vi "LCD Test.vi"() -> ()   [LabVIEW 2017]
panel:
  in  "stop":bool
  in  "String":string
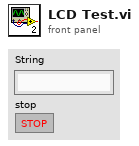
[diagram p1: front panel]
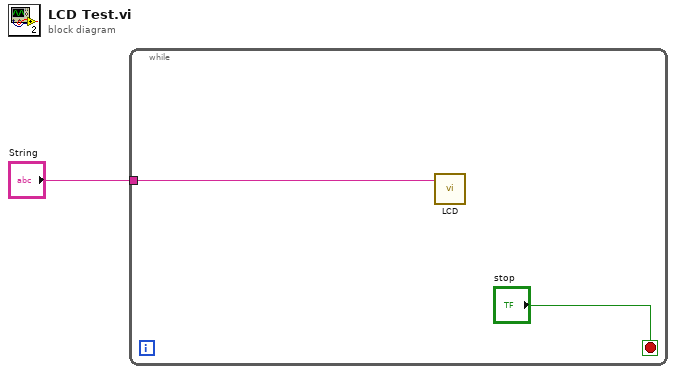
[diagram p0: block diagram]
diagram:
  n1 = while {
    tunnel: "String" -> [w2]
    stop <- "stop" stop-if-true
    n2 = call "LCD.vi"("String"=w2) -> ()  [unwired: 11 in]
  }
